vi "CounterView.vi"() -> ()   [LabVIEW 2013]
uses:
  Singleton.lvclass/Singleton.lvclass/Singleton.ctl
  Data.lvclass/Data.lvclass/Data.ctl
  Singleton.lvclass/ReadDataVariant.vi
  Singleton.lvclass/Constructor.vi
  Data.lvclass/Data.lvclass
panel:
  out "Counter":i32
  # "我是計數查看器"
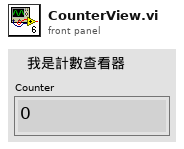
[diagram p1: front panel]
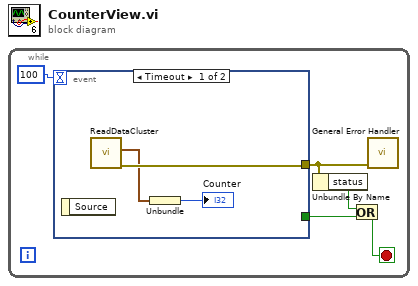
[diagram p0: block diagram]
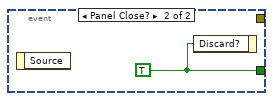
[diagram p2: hidden frame]
diagram:
  n1 = while {
    stop <- w3 stop-if-true
    n2 = event shown="[0] Timeout" {
      selector: _ -> [_ _]
      dyn-events: _ -> [_ _]
      timeout: 100 -> [_ _]
      tunnel: [_ w9] -> w4
      tunnel: [w8 _] -> w2
      event Timeout {
        n3 = event-data() -> ()  [unwired: 1 in, 1 out]
        n4 = call "ReadDataCluster.vi"() -> ("error out"=w8:errorcluster, "DataCluster"=w7:cluster{"CounterNum":i32})  [unwired: 10 in]
        n5 = Unbundle(w7) -> ("CounterNum"=→"Counter":i32)
      }
      event Panel Close? {
        w9 = TRUE
        n6 = event-data() -> ()  [unwired: 1 in, 1 out]
        n7 = event-data("Discard?"=w9) -> ()  [unwired: 1 in, 1 out]
      }
    }
    n8 = Unbundle By Name(w2) -> ("status"=w1:bool)
    n9 = Or(x=w1, y=w4) -> (x .or. y?=w3:bool)
    n10 = call <vilib>:"General Error Handler.vi"("error in (no error)"=w2) -> ()  [unwired: 10 in, 5 out]
  }
